vi "PM100D_Initial.vi"(4 "error in":errorcluster, 7 "VISA in":refnum<visa-resource-name>="USB0::0x1313::0x8078::P0027168::INSTR") -> (0 "error out":errorcluster, 1 "Sensor Flags":bool[](array[boolean]), 2 "IDN String":string, 3 "VISA out":refnum<visa-resource-name>)   [LabVIEW 2014]
panel:
  out "Sensor SN":string
  out "Sensor Name":string
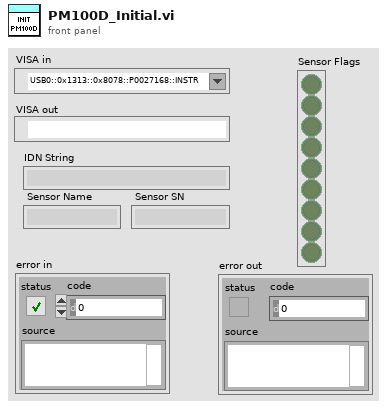
[diagram p1: front panel]
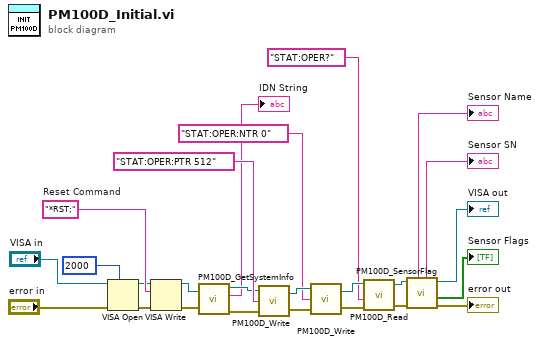
[diagram p0: block diagram]
diagram:
  w6 = "*RST;"  # Reset Command
  n1 = VISA Open(timeout (0)=u32 2000 ("VISA Open timeout (0)"), error in (no error)="error in", VISA resource name="VISA in") -> (VISA resource name=w2:refnum<visa-resource-name>, error out=w5:errorcluster)  [unwired: 2 out]
  n2 = VISA Write(VISA resource name=w2, write buffer=w6, error in (no error)=w5) -> (VISA resource name out=w3:refnum<visa-resource-name>, error out=w4:errorcluster)  [unwired: 1 out]
  n3 = call "PM100D_GetSystemInfo.vi"("VISA in"=w3, "error in"=w4) -> ("VISA out"=w21:refnum<visa-resource-name>, "Instrument"=→"IDN String":string, "error out"=w19:errorcluster)  [unwired: 1 out]
  n4 = call "PM100D_Write.vi"("error in (no error)"=w19, "Command"="STAT:OPER:PTR 512", "VISA in"=w21) -> ("error out"=w18:errorcluster, "VISA out"=w20:refnum<visa-resource-name>)
  n5 = call "PM100D_Write.vi"("error in (no error)"=w18, "Command"="STAT:OPER:NTR 0", "VISA in"=w20) -> ("error out"=w14:errorcluster, "VISA out"=w16:refnum<visa-resource-name>)
  n6 = call "PM100D_Read.vi"("error in (no error)"=w14, "Command"="STAT:OPER?", "VISA in"=w16) -> ("error out"=w10:errorcluster, "VISA out"=w11:refnum<visa-resource-name>)  [unwired: 1 in, 1 out]
  n7 = call "PM100D_SensorFlag.vi"("error in (no error)"=w10, "VISA in"=w11) -> ("error out"=→"error out":errorcluster, "flags"=→"Sensor Flags":bool[], "VISA out"=→"VISA out":refnum<visa-resource-name>, "sn"=→"Sensor SN":string, "name"=→"Sensor Name":string)  [unwired: 2 in, 3 out]
